vi "Create from SFTP Directory.vi"(8 "Error In":errorcluster, 11 "SFTP Directory In":refnum<class "SFTP Directory.lvclass">) -> (0 "Error Out":errorcluster, 2 "SFTP Attributes":refnum<class "SFTP Attributes.lvclass">, 3 "SFTP Directory Out":refnum<class "SFTP Directory.lvclass">)   [LabVIEW 2018, in "Toolkit.lvlib" / "SFTP Attributes.lvclass"]
uses:
  SFTP Attributes.lvclass
  SFTP Directory/SFTP Directory.lvclass
  SFTP Directory/SFTP Directory.lvclass/SFTP Directory.ctl
  SFTP/SFTP.lvclass/SFTP.ctl
  Session/Session.lvclass/Session.ctl
  SSH/SSH.lvclass
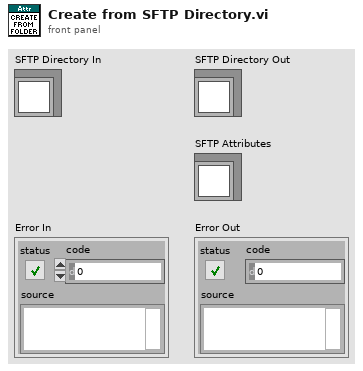
[diagram p1: front panel]
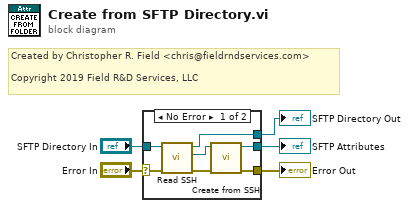
[diagram p0: block diagram]
diagram:
  # "Created by Christopher R. Field <chris@fieldrndservices.com>\n\nCopyright 2019 Field R&D Services, LLC"
  n1 = case shown="No Error" "Error In" {
    selector: "Error In" -> [w7 w14]
    tunnel: [w11 w14] -> w4
    tunnel: [w12 _] -> w3
    tunnel: "SFTP Directory In" -> [w10 w13]
    tunnel: [w6 w13] -> w1
    frame No Error {
      n2 = call "Read SSH.vi"("Error In"=w7, "SFTP Directory In"=w10) -> ("Error Out"=w8:errorcluster, "SSH"=w9:refnum<class "SSH.lvclass">, "SFTP Directory Out"=w6:refnum<class "SFTP Directory.lvclass">)  [unwired: 7 in]
      n3 = call "Create from SSH.vi"("Error In"=w8, "SSH"=w9) -> ("Error Out"=w11:errorcluster, "SFTP Attributes"=w12:refnum<class "SFTP Attributes.lvclass">)  [unwired: 8 in]
    }
    frame Error {
    }
  }
  "Error Out" <- w4
  "SFTP Attributes" <- w3
  "SFTP Directory Out" <- w1
